vi "4110_Create I Chans.vi"(5 "Device Ref in":T1 format="%.0x", 7 "# of I Channels to Add?":i16, 8 "error in":errorcluster, 9 "sense":T2=1008 caption="sense (out)" items=["Local"=1008, "Remote"=1009], 10 "Voltage Limit":dbl, 11 "Init Value":dbl) -> (0 "error out":errorcluster)   [LabVIEW 2018, in "NI PXI-4110 Programmable Power Supply Custom Device.lvlib"]
uses:
  NI PXI-4110 Programmable Power Supply Custom Device.lvlib
  <instrlib>/niDCPower/nidcpower.llb/niDCPower Sense.ctl
  <vilib>/NI Veristand/Custom Device API/Custom Device Item Ref.ctl
  <vilib>/NI Veristand/Custom Device API/Custom Device Channel.ctl
  <vilib>/NI Veristand/Custom Device API/Custom Device Channel Type.ctl
  4110_Global.vi
  <vilib>/NI Veristand/Custom Device API/Get Item Property (U16).vi
  <vilib>/NI Veristand/Custom Device API/Set Item Property (U16).vi
  <vilib>/NI VeriStand/Custom Device API/Custom Device API.lvlib
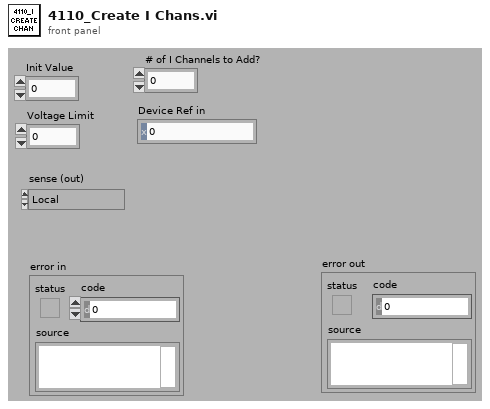
[diagram p1: front panel]
types:
  T1 = typedef "Custom Device API.lvlib/Custom Device Item Ref.ctl" = u64
  T2 = typedef "niDCPower Sense.ctl" = i32
  T3 = typedef "Custom Device API.lvlib/Custom Device Channel.ctl" = cluster{"Type":T4, "Units":string, "Default Value":dbl, "Faultable":bool, "Scalable":bool}
  T4 = typedef "Custom Device API.lvlib/Custom Device Channel Type.ctl" = enum16{"Input", "Output"}
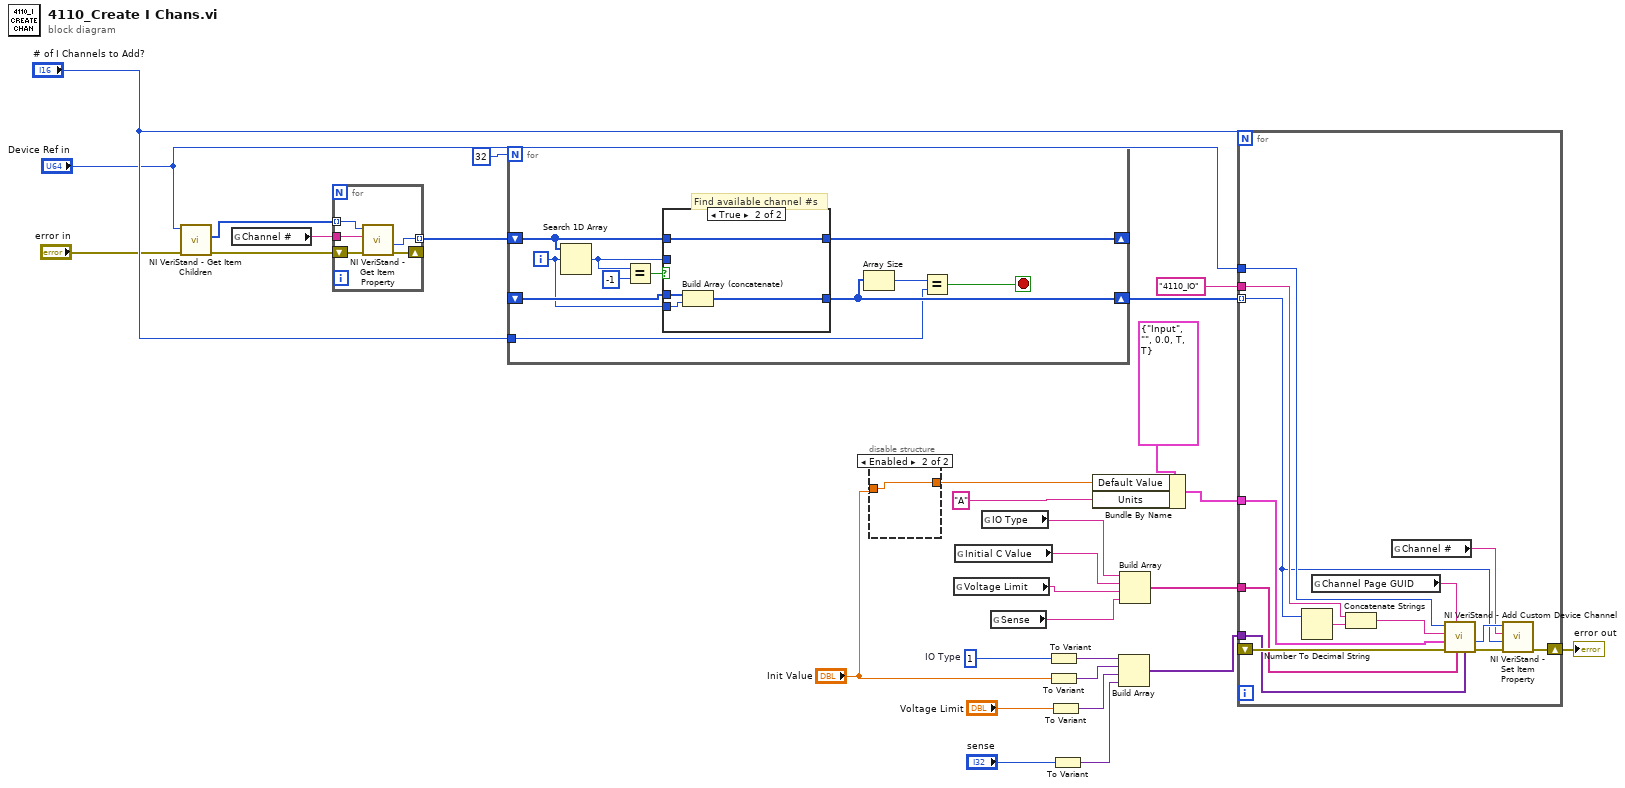
[diagram p0: block diagram]
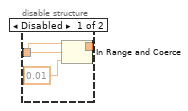
[diagram p2: hidden frame]
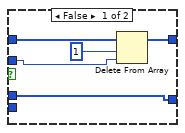
[diagram p3: hidden frame]
diagram:
  w6 = u16 1  # IO Type
  n1 = call <vilib>:"NI VeriStand - Get Item Children.vi"("error in (no error)"="error in", "Item Ref in"="Device Ref in") -> ("error out"=w19:errorcluster, "Child Refs"=w20:T1[])  [unwired: 6 in, 2 out]
  n2 = global read "4110_Global.vi" "Channel #"() -> (w11:string)
  n3 = for {
    tunnel: w20 -> [w34] mode=indexing
    shift-right: [w31] -> _
    shift-left: w19 -> [w33]
    tunnel: w11 -> [w32]
    tunnel: [w30] -> w18 mode=indexing
    n4 = call-poly <vilib>:"NI VeriStand - Get Item Property.vi"("error in (no error)"=w33, "Property Name"=w32, "Item Ref in"=w34) -> ("error out"=w31:errorcluster, "Value"=w30:u16)  [unwired: 5 in, 2 out]
  }
  n5 = for {
    N: 32 -> [_]
    shift-right: [w38] -> w17
    shift-left: _ -> [w43]
    shift-right: [w39] -> _
    shift-left: w18 -> [w41]
    tunnel: "# of I Channels to Add?" -> [w36]
    i -> [w42]
    stop <- w35 stop-if-true
    # "Find available channel #s"
    n6 = Search 1D Array(1D array=w41, element=w42) -> (index of element=w40:i32)  [unwired: 1 in]
    n7 = Equal?(x=w40, y=-1) -> (x = y?=w44:bool)
    n8 = case shown="True" w44 {
      tunnel: w43 -> [w50 w54]
      tunnel: [w50 w53] -> w38
      tunnel: w42 -> [_ w52]
      tunnel: w41 -> [w49 w51]
      tunnel: w40 -> [w47 _]
      tunnel: [w46 w51] -> w39
      frame False {
        n9 = Delete From Array(array=w49, length=1, index=w47) -> (array with subset deleted=w46:u16[])  [unwired: 1 out]
      }
      frame True {
        n10 = Build Array (concatenate)(w54, w52) -> (w53:i32[])
      }
    }
    n11 = Array Size(array=w38) -> (size(s)=w37:i32)
    n12 = Equal?(x=w37, y=w36) -> (x = y?=w35:bool)
  }
  n13 = disable-structure shown="Enabled" {
    disable-tunnel: "Init Value" -> [w56 w58]
    disable-tunnel: [w55 w58] -> w1
    frame Disabled {
      n14 = In Range and Coerce(upper limit=w56, x=w56, lower limit=0.01 ("Default Value")) -> (coerced(x)=w55:dbl)  [unwired: 1 out]
    }
    frame Enabled {
    }
  }
  n15 = global read "4110_Global.vi" "Voltage Limit"() -> (w8:string)
  n16 = global read "4110_Global.vi" "Initial C Value"() -> (w9:string)
  n17 = global read "4110_Global.vi" "IO Type"() -> (w10:string)
  n18 = global read "4110_Global.vi" "Sense"() -> (w7:string)
  n19 = To Variant(anything=w6) -> (Variant=w24:variant)
  n20 = To Variant(anything="Init Value") -> (Variant=w25:variant)
  n21 = To Variant(anything="Voltage Limit") -> (Variant=w26:variant)
  n22 = To Variant(anything="sense") -> (Variant=w27:variant)
  n23 = Bundle By Name(cluster=T3 {"Type"=enum."Input", "Units"="", "Default Value"=0.0, "Faultable"=TRUE, "Scalable"=TRUE} ("Channel"), "Default Value"=w1, "Units"="A") -> (w15:T3)
  n24 = Build Array(w24, w25, w26, w27) -> (w28:variant[])
  n25 = Build Array(w10, w9, w8, w7) -> (w29:string[])
  n26 = for {
    N: "# of I Channels to Add?" -> [_]
    shift-right: [w65] -> w22
    shift-left: _ -> [w72]
    tunnel: w15 -> [w71]
    tunnel: "Device Ref in" -> [w70]
    tunnel: "4110_IO" -> [w69]
    tunnel: w28 -> [w63]
    tunnel: w29 -> [w62]
    tunnel: w17 -> [w61] mode=indexing
    n27 = Number To Decimal String(number=w61) -> (decimal integer string=w68:string)  [unwired: 1 in]
    n28 = global read "4110_Global.vi" "Channel Page GUID"() -> (w59:string)
    n29 = Concatenate Strings(w69, w68) -> (w67:string)
    n30 = global read "4110_Global.vi" "Channel #"() -> (w60:string)
    n31 = call <vilib>:"NI VeriStand - Add Custom Device Channel.vi"("Property Values"=w63, "Property names"=w62, "GUID (Default Channel)"=w59, "error in (no error)"=w72, "Channel"=w71, "Channel Name"=w67, "Parent Ref in"=w70) -> ("error out"=w66:errorcluster, "Channel Ref"=w64:T1)  [unwired: 1 in, 2 out]
    n32 = call-poly <vilib>:"NI VeriStand - Set Item Property.vi"("error in (no error)"=w66, "Value"=w61, "Property Name"=w60, "Item Ref in"=w64) -> ("error out"=w65:errorcluster)  [unwired: 5 in, 2 out]
  }
  "error out" <- w22
